vi "Caller.vi"(0 "Divide in":refnum<class "Divide.lvclass">, 5 "Sub Panel":refnum<vi>, 7 "State":refnum<user-event>, 9 "Class Data":refnum<user-event>, 11 "Error In":errorcluster) -> (4 "Divide out":refnum<class "Divide.lvclass">, 15 "Error Out":errorcluster)   [LabVIEW 2023, in "Divide.lvclass"]
doc: "The VI asynchronously calls the Operation UI method of the division operation."
uses:
  Divide.lvclass
  C:/Users/Ancy.Augustin/Downloads/LVOOPS DVR/LVOOPS DVR/Classes/Arithemtic Operation/Arithemetic Operation.lvclass
  Arithemtic Operation/Arithemetic Operation.lvclass
  Operation UI.vi
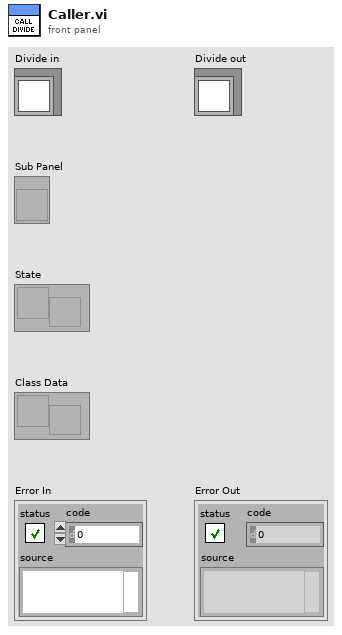
[diagram p1: front panel]
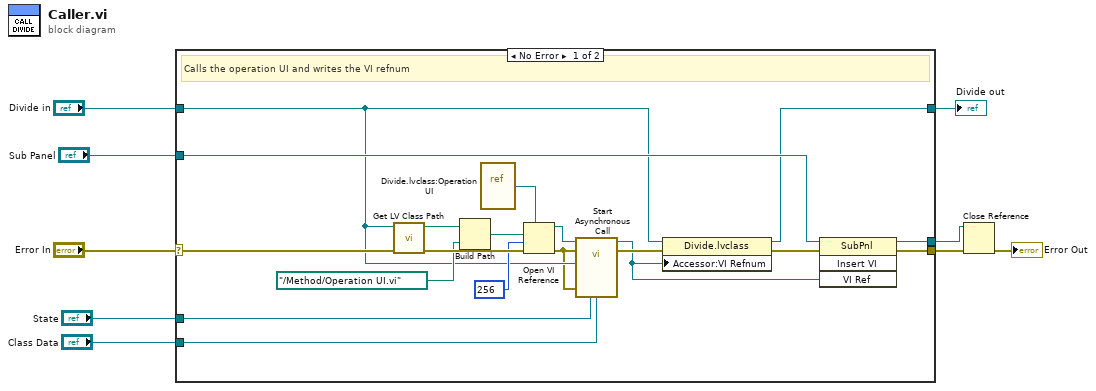
[diagram p0: block diagram]
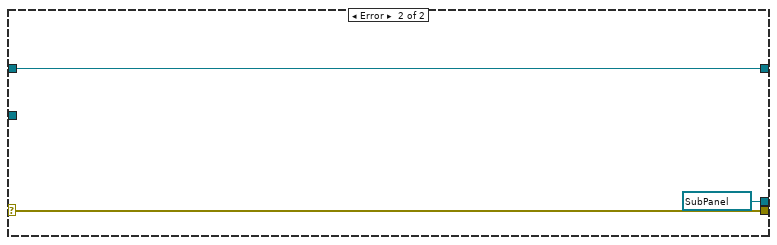
[diagram p2: hidden frame]
diagram:
  n1 = case shown="No Error" "Error In" {
    selector: "Error In" -> [w21 w31]
    tunnel: [w20 w31] -> w8
    tunnel: [w14 w30] -> w6
    tunnel: "Divide in" -> [w12 w30]
    tunnel: "State" -> [w19 _]
    tunnel: "Class Data" -> [w18 _]
    tunnel: "Sub Panel" -> [w17 _]
    tunnel: [w13 refnum<vi> refnum ("Sub Panel")] -> w1
    frame No Error {
      # "Calls the operation UI and writes the VI refnum"
      n2 = call <vilib>:"Get LV Class Path.vi"("error in (no error)"=w21, "object"=w12) -> ("error out"=w28:errorcluster, "class path"=w27:path)  [unwired: 8 in]
      n3 = Build Path(base path=w27, name or relative path=path "../Method/Operation UI.vi") -> (appended path=w11:path)
      n4 = vi-ref "Divide.lvclass:Operation UI.vi"() -> (w22:refnum<vi>)
      n5 = Open VI Reference(type specifier VI Refnum (for type only)=w22, vi path=w11, options=256, error in (no error)=w28) -> (vi reference=w25:refnum<vi>, error out=w10:errorcluster)  [unwired: 2 in]
      n6 = call-by-ref "Start Asynchronous Call"(reference=w25, error in=w10, "Divide in"=w12, "Error In"=w10, "user event out 2"=w19, "user event out"=w18) -> (reference out=w15:refnum<vi>, error out=w24:errorcluster)  [unwired: 9 in, 3 out]
      n7 = property class="Divide.lvclass"(reference=w12, error in=w24, "Accessor:VI Refnum"=w15) -> (reference out=w14:refnum<class "Divide.lvclass">, error out=w16:errorcluster)
      n8 = invoke on="Invoke Node" class="SubPnl" method="Insert VI"(reference=w17, error in=w16, "VI Ref"=w15) -> (reference out=w13:refnum<vi>, error out=w20:errorcluster)  [unwired: 1 in, 2 out]
    }
    frame Error {
    }
  }
  "Divide out" <- w6
  n9 = Close Reference(reference=w1, error in (no error)=w8) -> (error out=→"Error Out":errorcluster)
